vi "Queues FGV.vi"(11 "Enum":T2) -> (3 "Queues":T1)   [LabVIEW 2014]
uses:
  set_get.ctl
  CMD UI enum.ctl
  CMD Report enum.ctl
  CMD DA enum.ctl
  CMD DAQ enum.ctl
  CMD LOG enum.ctl
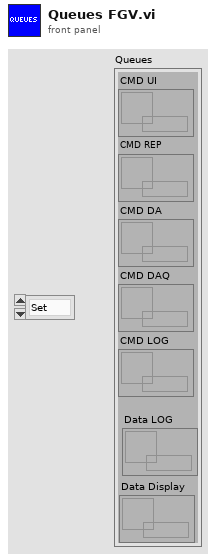
[diagram p1: front panel]
types:
  T1 = cluster{"CMD UI":refnum<queue>, "CMD REP":refnum<queue>, "CMD DA":refnum<queue>, "CMD DAQ":refnum<queue>, "CMD LOG":refnum<queue>, "Data LOG":refnum<queue>, "Data Display":refnum<queue>}
  T2 = typedef "set_get.ctl" = enum16{"Set", "Get"}
  T3 = typedef "CMD LOG enum.ctl" = enum16{"Start Log", "Log", "Stop Log", "Exit"}
  T4 = typedef "CMD DAQ enum.ctl" = enum16{"Init DAQ", "Init Read From File", "DAQ", "Read From File", "Stop DAQ", "Stop Read From File", "Exit"}
  T5 = typedef "CMD DA enum.ctl" = enum16{"Wait", "Analyze", "Meta Analyze", "Exit"}
  T6 = typedef "CMD Report enum.ctl" = enum16{"Create Report", "Exit"}
  T7 = typedef "CMD UI enum.ctl" = enum16{"Init all", "Update Patient Info", "Update Analyzed", "Create Report", "Analyze Data", "Start DAQ", "Start Read", "LOG Data", "Stop LOG Data", "Stop DAQ", "Stop Read", "EXIT"}
  T8 = cluster{"queue out":refnum<queue>, "queue out":refnum<queue>, "queue out":refnum<queue>, "queue out":refnum<queue>, "queue out":refnum<queue>, "queue out":refnum<queue>, "queue out":refnum<queue>}
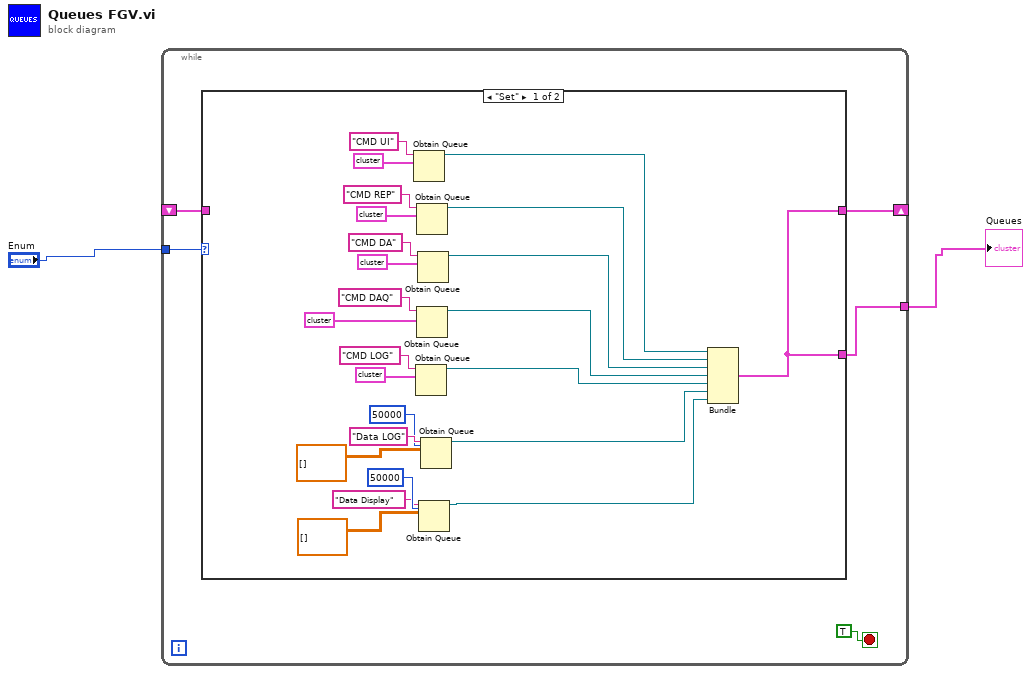
[diagram p0: block diagram]
diagram:
  n1 = while {
    tunnel: "Enum" -> [w6]
    shift-right: [w5] -> _
    shift-left: _ -> [w4]
    tunnel: [w3] -> w1
    stop <- TRUE stop-if-true
    n2 = case shown="\"Set\"" w6 {
      tunnel: [w26 w32] -> w3
      tunnel: [w26 w32] -> w5
      tunnel: w4 -> [_ w32]
      frame "Set" {
        n3 = Obtain Queue(name (unnamed)="CMD UI", element data type=cluster{variant, T7} {variant, enum."Start DAQ"}) -> (queue out=w27:refnum<queue>)  [unwired: 3 in, 2 out]
        n4 = Obtain Queue(name (unnamed)="CMD LOG", element data type=cluster{variant, T3} {variant, enum."Start Log"}) -> (queue out=w9:refnum<queue>)  [unwired: 3 in, 2 out]
        n5 = Obtain Queue(name (unnamed)="CMD REP", element data type=cluster{variant, T6} {variant, enum."Create Report"}) -> (queue out=w12:refnum<queue>)  [unwired: 3 in, 2 out]
        n6 = Obtain Queue(name (unnamed)="CMD DAQ", element data type=cluster{variant, T4} {variant, enum."Init DAQ"}) -> (queue out=w10:refnum<queue>)  [unwired: 3 in, 2 out]
        n7 = Obtain Queue(name (unnamed)="CMD DA", element data type=cluster{variant, T5} {variant, enum."Wait"}) -> (queue out=w11:refnum<queue>)  [unwired: 3 in, 2 out]
        n8 = Obtain Queue(max queue size (-1, unlimited)=50000, name (unnamed)="Data Display", element data type=dbl[][] []) -> (queue out=w13:refnum<queue>)  [unwired: 2 in, 2 out]
        n9 = Obtain Queue(max queue size (-1, unlimited)=50000, name (unnamed)="Data LOG", element data type=dbl[][] []) -> (queue out=w14:refnum<queue>)  [unwired: 2 in, 2 out]
        n10 = Bundle("queue out"=w27, "queue out"=w12, "queue out"=w11, "queue out"=w10, "queue out"=w9, "queue out"=w14, "queue out"=w13) -> (w26:T8)  [unwired: 1 in]
      }
      frame "Get", Default {
      }
    }
  }
  "Queues" <- w1
